vi "NI-9870_SoftPanel.vi"(3 "NI-9870 in Slot:":string="1") -> ()   [LabVIEW 2016]
uses:
  HelperSubVIs/GlobalControlVariables.vi
panel:
  in  "Set":bool
  in  "Channel":string(combo)="CH1"
  in  "Clear":bool
  in  "Baudrate":string(combo)="9600"
  out "ExitModule":bool=TRUE
  out "Received":string
  in  "Message":string
  in  "Transmit":bool
  in  "ExitButton":bool
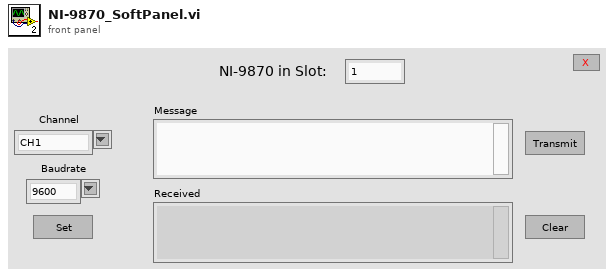
[diagram p1: front panel]
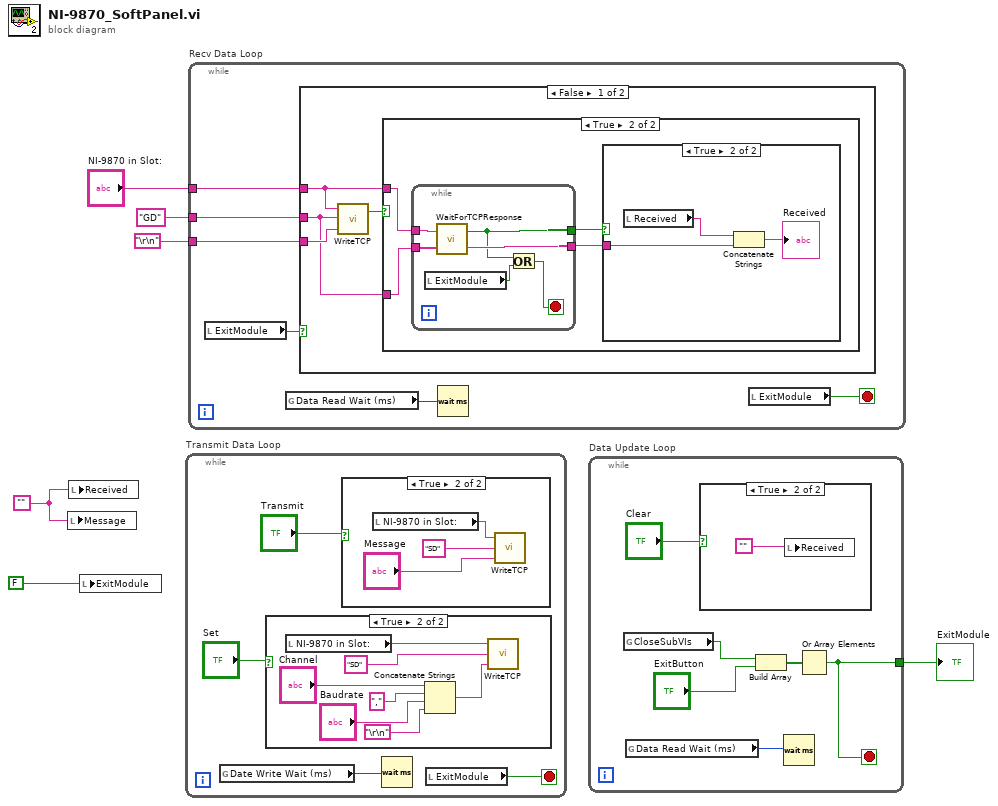
[diagram p0: block diagram]
diagram:
  w1 = ""
  n1 = local write "Message"(w1) -> ()
  n2 = local write "Received"(w1) -> ()
  n3 = local write "ExitModule"(FALSE) -> ()
  n4 = while "Transmit Data Loop" {
    stop <- w9 stop-if-true
    n5 = global read "GlobalControlVariables.vi" "Date Write Wait (ms)"() -> (w8:u32)
    n6 = case shown="True" "Set" {
      frame False {
      }
      frame True {
        n7 = local read "NI-9870 in Slot:"() -> (w17:string)
        n8 = Concatenate Strings("Channel", ",", "Baudrate", "\r\n") -> (w11:string)
        n9 = call "WriteTCP.vi"("Data"=w11, "Action"="SD", "Module Slot"=w17) -> ()  [unwired: 2 out]
      }
    }
    n10 = case shown="True" "Transmit" {
      frame False {
      }
      frame True {
        n11 = local read "NI-9870 in Slot:"() -> (w19:string)
        n12 = call "WriteTCP.vi"("Data"="Message", "Action"="SD", "Module Slot"=w19) -> ()  [unwired: 2 out]
      }
    }
    n13 = Wait (ms)(milliseconds to wait=w8) -> ()  [unwired: 1 out]
    n14 = local read "ExitModule"() -> (w9:bool)
  }
  n15 = while "Recv Data Loop" {
    tunnel: "NI-9870 in Slot:" -> [w25]
    tunnel: "\r\n" -> [w23]
    tunnel: "GD" -> [w22]
    stop <- w26 stop-if-true
    n16 = local read "ExitModule"() -> (w21:bool)
    n17 = global read "GlobalControlVariables.vi" "Data Read Wait (ms)"() -> (w24:u32)
    n18 = case shown="False" w21 {
      tunnel: w25 -> [w29 _]
      tunnel: w23 -> [w28 _]
      tunnel: w22 -> [w27 _]
      frame False {
        n19 = call "WriteTCP.vi"("Data"=w28, "Action"=w27, "Module Slot"=w29) -> ("Sent"=w30:bool)  [unwired: 1 out]
        n20 = case shown="True" w30 {
          tunnel: w29 -> [_ w33]
          tunnel: w27 -> [_ w32]
          frame False {
          }
          frame True {
            n21 = while {
              tunnel: [w35] -> w34
              tunnel: w33 -> [w40]
              tunnel: w32 -> [w39]
              tunnel: [w38] -> w31
              stop <- w36 stop-if-true
              n22 = local read "ExitModule"() -> (w37:bool)
              n23 = call "WaitForTCPResponse.vi"("Action"=w39, "Module Slot"=w40) -> ("Received Data"=w38:string, "Ready"=w35:bool)
              n24 = Or(x=w35, y=w37) -> (x .or. y?=w36:bool)
            }
            n25 = case shown="True" w34 {
              tunnel: w31 -> [_ w41]
              frame False {
              }
              frame True {
                n26 = local read "Received"() -> (w42:string)
                n27 = Concatenate Strings(w42, w41) -> (→"Received":string)
              }
            }
          }
        }
      }
      frame True {
      }
    }
    n28 = Wait (ms)(milliseconds to wait=w24) -> ()  [unwired: 1 out]
    n29 = local read "ExitModule"() -> (w26:bool)
  }
  n30 = while "Data Update Loop" {
    tunnel: [w45] -> w6
    stop <- w45 stop-if-true
    n31 = global read "GlobalControlVariables.vi" "CloseSubVIs"() -> (w46:bool)
    n32 = global read "GlobalControlVariables.vi" "Data Read Wait (ms)"() -> (w49:u32)
    n33 = case shown="True" "Clear" {
      frame False {
      }
      frame True {
        n34 = local write "Received"("") -> ()
      }
    }
    n35 = Build Array(w46, "ExitButton") -> (w48:bool[])
    n36 = Wait (ms)(milliseconds to wait=w49) -> ()  [unwired: 1 out]
    n37 = Or Array Elements(Boolean array=w48) -> (logical OR=w45:bool)
  }
  "ExitModule" <- w6
